vi "MeaCurr8341.vi"(10 "测试类型":u16(ring) items=["DCV", "ACV", "DCI", "ACI", "OHM", "RST", "CAP", "FRQ", "AUTO"], 11 "VISA名称":refnum<visa-resource-name>="COM1") -> (0 "错误输出":errorcluster, 2 "数值":dbl format="%#_3g")   [LabVIEW 2013]
uses:
  <vilib>/Instr/_visa.llb/VISA Flush IO Buffer Mask.ctl
  <vilib>/Instr/_visa.llb/VISA Configure Serial Port (Instr).vi
panel:
  out "响应":string
  in  "串口设置":T1={"波特率"=9600, "数据比特"=8, "奇偶"=enum."None", "停止位"=10, "流控制"=0} {"流控制" items=["无"=0, "XON/XOFF"=1, "RTS/CTS"=2, "DTR/DSR"=4]; "停止位" items=["1.0"=10, "1.5"=15, "2.0"=20]; "数据比特" min=5 max=8 step=1; "波特率" items=["75"=75, "110"=110, "134"=134, "150"=150, "300"=300, "600"=600, "1200"=1200, "1800"=1800, "2400"=2400, "4800"=4800, "7200"=7200, "9600"=9600, "14400"=14400, "19200"=19200, "28800"=28800, "38400"=38400, "56000"=56000, "57600"=57600, "115200"=115200, "128000"=128000, "230400"=230400]}
  in  "读取前延时":u32=600
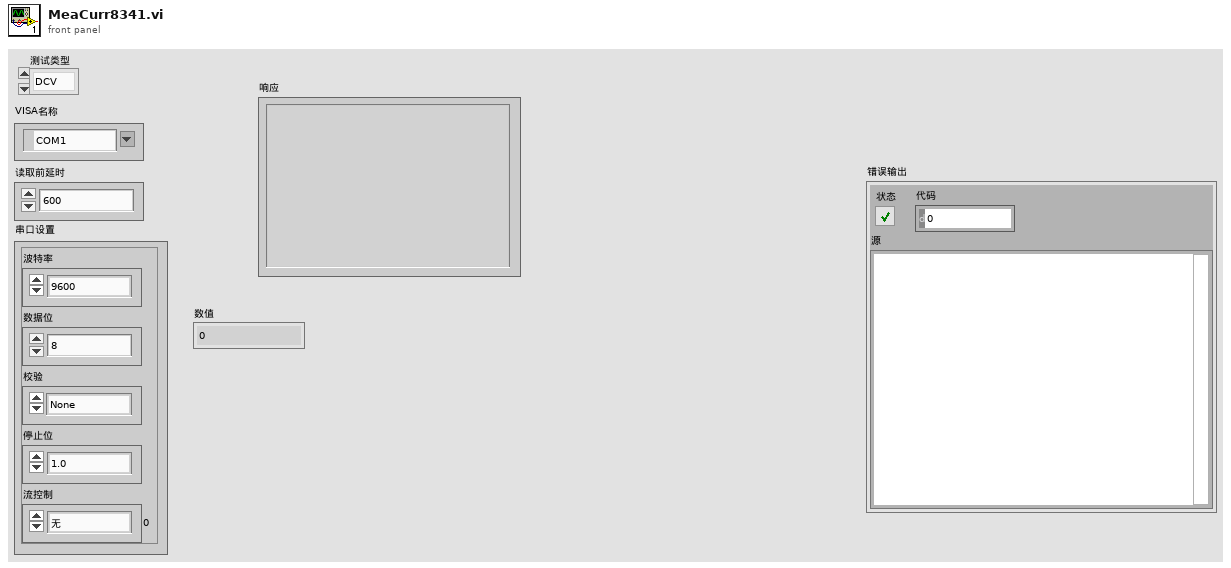
[diagram p1: front panel]
types:
  T1 = cluster{"波特率":u32, "数据比特":u16, "奇偶":enum16{"None", "Odd", "Even", "Mark", "Space"}, "停止位":u16, "流控制":u16}
  T2 = typedef "VISA Flush IO Buffer Mask.ctl" = u16
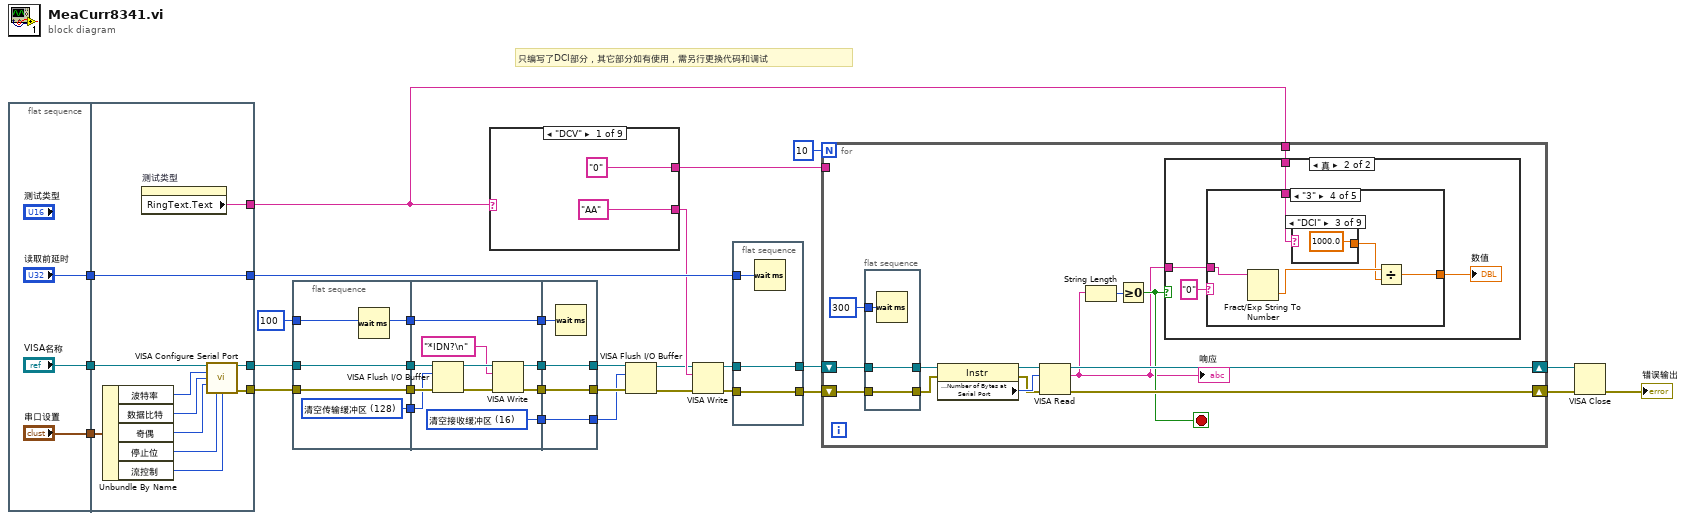
[diagram p0: block diagram]
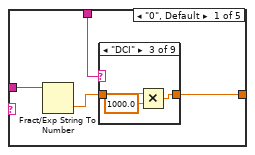
[diagram p3: hidden frame]
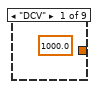
[diagram p4: hidden frame]
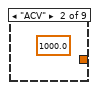
[diagram p5: hidden frame]
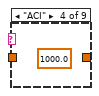
[diagram p6: hidden frame]
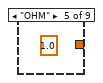
[diagram p7: hidden frame]
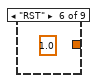
[diagram p8: hidden frame]
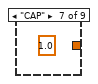
[diagram p9: hidden frame]
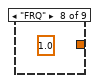
[diagram p10: hidden frame]
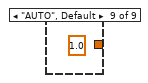
[diagram p11: hidden frame]
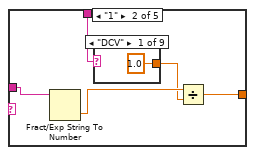
[diagram p12: hidden frame]
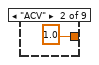
[diagram p13: hidden frame]
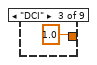
[diagram p14: hidden frame]
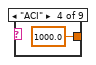
[diagram p15: hidden frame]
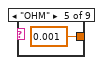
[diagram p16: hidden frame]
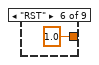
[diagram p17: hidden frame]
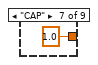
[diagram p18: hidden frame]
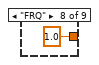
[diagram p19: hidden frame]
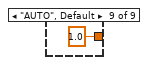
[diagram p20: hidden frame]
diagram:
  # "只编写了DCI部分，其它部分如有使用，需另行更换代码和调试"
  n1 = flat-sequence {
    tunnel: ["VISA名称"] -> w9
    tunnel: ["读取前延时"] -> w8
    tunnel: ["串口设置"] -> w7
    tunnel: [w45] -> w27
    tunnel: w9 -> [w38]
    tunnel: w8 -> [w45]
    tunnel: w7 -> [w39]
    tunnel: [w37] -> w5
    tunnel: [w36] -> w3
    tunnel: [w35] -> w2
    frame #0 {
    }
    frame #1 {
      n2 = Unbundle By Name(w39) -> ("波特率"=w40:u32, "数据比特"=w41:u16, "奇偶"=w42:enum16{"None", "Odd", "Even", "Mark", "Space"}, "停止位"=w43:u16, "流控制"=w44:u16)
      n3 = property on="测试类型" class="Ring (严格)"() -> ("RingText.Text"=w35:string)  [unwired: 2 in, 2 out]
      n4 = call-poly "VISA Configure Serial Port"("VISA resource name"=w38, "baud rate (9600)"=w40, "data bits (8)"=w41, "parity (0:none)"=w42, "stop bits (10: 1 bit)"=w43, "flow control (0:none)"=w44) -> ("VISA resource name out"=w37:refnum<visa-resource-name>, "error out"=w36:errorcluster)  [unwired: 3 in, 5 out]
    }
  }
  n5 = flat-sequence {
    tunnel: u32 100 ("读取前延时(ms)") -> [w49]
    tunnel: [w49] -> w18
    tunnel: [w48] -> w6
    tunnel: w5 -> [w48]
    tunnel: [w47] -> w4
    tunnel: w3 -> [w47]
    tunnel: [w46] -> w1
    tunnel: [w55] -> w21
    tunnel: [w56] -> w20
    tunnel: [w54] -> w19
    tunnel: w18 -> [w54]
    tunnel: [w53] -> w17
    tunnel: w6 -> [w52]
    tunnel: w4 -> [w51]
    tunnel: w1 -> [w50]
    tunnel: [w61] -> w14
    tunnel: [w62] -> w13
    tunnel: w21 -> [w62]
    tunnel: w20 -> [w61]
    tunnel: w19 -> [w63]
    tunnel: w17 -> [w60]
    tunnel: [w60] -> w12
    frame #0 {
      w46 = T2 128 items=["清空接收缓冲区"=16, "向设备写入传输缓冲区"=32, "清空接收缓冲区（无I/O）"=64, "清空传输缓冲区"=128] ("Mask")
      n6 = Wait (ms)(milliseconds to wait=w49) -> ()  [unwired: 1 out]
    }
    frame #1 {
      w53 = T2 16 items=["清空接收缓冲区"=16, "向设备写入传输缓冲区"=32, "清空接收缓冲区（无I/O）"=64, "清空传输缓冲区"=128] ("Mask")
      n7 = VISA Flush I/O Buffer(VISA resource name=w52, mask (16)=w50, error in (no error)=w51) -> (VISA resource name out=w58:refnum<visa-resource-name>, error out=w59:errorcluster)
      n8 = VISA Write(VISA resource name=w58, write buffer="*IDN?\n" ("写入缓冲区"), error in (no error)=w59) -> (VISA resource name out=w56:refnum<visa-resource-name>, error out=w55:errorcluster)  [unwired: 1 out]
    }
    frame #2 {
      n9 = Wait (ms)(milliseconds to wait=w63) -> ()  [unwired: 1 out]
    }
  }
  n10 = case shown="\"DCV\"" w2 {
    tunnel: ["AA" ("Command") "BB" ("Command") "MEAS:CURR:DC? 5e\n" "DD" ("Command") "EE" ("Command") "FF" ("Command") "GG" ("Command") "HH" ("Command") "MM" ("Command")] -> w26
    tunnel: ["0" ("Command") "1" ("Command") "3" ("Command") "4" ("Command") "6" ("Command") "F" ("Command") "7" ("Command") "8" ("Command") "M" ("Command")] -> w25
    frame "DCV" {
    }
    frame "ACV" {
    }
    frame "DCI" {
      n11 = local write "数值"(0.0 ("数值")) -> ()
    }
    frame "ACI" {
    }
    frame "OHM" {
    }
    frame "RST" {
    }
    frame "CAP" {
    }
    frame "FRQ" {
    }
    frame "AUTO", Default {
    }
  }
  n12 = VISA Flush I/O Buffer(VISA resource name=w14, mask (16)=w12, error in (no error)=w13) -> (VISA resource name out=w10:refnum<visa-resource-name>, error out=w11:errorcluster)
  n13 = VISA Write(VISA resource name=w10, write buffer=w26, error in (no error)=w11) -> (VISA resource name out=w16:refnum<visa-resource-name>, error out=w15:errorcluster)  [unwired: 1 out]
  n14 = flat-sequence {
    tunnel: [w83] -> w29
    tunnel: [w84] -> w28
    tunnel: w27 -> [w85]
    tunnel: w16 -> [w84]
    tunnel: w15 -> [w83]
    frame #0 {
      n15 = Wait (ms)(milliseconds to wait=w85) -> ()  [unwired: 1 out]
    }
  }
  n16 = for {
    N: 10 -> [_]
    tunnel: w25 -> [_]
    tunnel: w2 -> [w96]
    shift-right: [w98] -> w30
    shift-left: w28 -> [w95]
    shift-right: [w99] -> w31
    shift-left: w29 -> [w93]
    stop <- w90 stop-if-true
    n17 = flat-sequence {
      tunnel: w93 -> [w101]
      tunnel: [w101] -> w92
      tunnel: w95 -> [w100]
      tunnel: [w100] -> w94
      tunnel: u32 300 ("读取前延时(ms)") -> [w102]
      frame #0 {
        n18 = Wait (ms)(milliseconds to wait=w102) -> ()  [unwired: 1 out]
      }
    }
    n19 = property class="Instr"(reference=w94, error in=w92) -> (reference out=w89:refnum<visa-resource-name>, error out=w88:errorcluster, "Serial Settings:Number of Bytes at Serial Port"=w97:u32)
    n20 = VISA Read(VISA resource name=w89, byte count=w97, error in (no error)=w88) -> (VISA resource name out=w98:refnum<visa-resource-name>, read buffer=w86:string, error out=w99:errorcluster)  [unwired: 1 out]
    "响应" <- w86
    n21 = String Length(string=w86) -> (length=w87:i32)
    n22 = Greater Or Equal To 0?(x=w87) -> (x >= 0?=w90:bool)
    n23 = case shown="真" w90 {
      tunnel: w86 -> [_ w103]
      tunnel: w96 -> [_ w106]
      frame False {
      }
      frame True {
        n24 = case shown="\"3\"" "0" {
          tunnel: w103 -> [w110 w118 w132 w146 w160]
          tunnel: w106 -> [w109 w117 w131 w145 w159]
          tunnel: [w108 w114 w128 w142 w156] -> w105
          frame "0", Default {
            n25 = Fract/Exp String To Number(string=w110) -> (number=w107:dbl)  [unwired: 3 in, 1 out]
            n26 = case shown="\"DCI\"" w109 {
              tunnel: [_ _ w111 _ _ _ _ _ _] -> w108
              tunnel: w107 -> [_ _ w113 _ _ _ _ _ _]
              frame "DCV" {
                (unwired) 1000.0
              }
              frame "ACV" {
                (unwired) 1000.0
              }
              frame "DCI" {
                n27 = Multiply(x=w113, y=1000.0) -> (x*y=w111:dbl)
              }
              frame "ACI" {
                (unwired) 1000.0
              }
              frame "OHM" {
                (unwired) 1.0
              }
              frame "RST" {
                (unwired) 1.0
              }
              frame "CAP" {
                (unwired) 1.0
              }
              frame "FRQ" {
                (unwired) 1.0
              }
              frame "AUTO", Default {
                (unwired) 1.0
              }
            }
          }
          frame "1" {
            n28 = Fract/Exp String To Number(string=w118) -> (number=w116:dbl)  [unwired: 3 in, 1 out]
            n29 = case shown="\"DCV\"" w117 {
              tunnel: [1.0 1.0 1.0 1000.0 0.001 1.0 1.0 1.0 1.0] -> w115
              frame "DCV" {
              }
              frame "ACV" {
              }
              frame "DCI" {
              }
              frame "ACI" {
              }
              frame "OHM" {
              }
              frame "RST" {
              }
              frame "CAP" {
              }
              frame "FRQ" {
              }
              frame "AUTO", Default {
              }
            }
            n30 = Divide(x=w116, y=w115) -> (x/y=w114:dbl)
          }
          frame "2" {
            n31 = Fract/Exp String To Number(string=w132) -> (number=w130:dbl)  [unwired: 3 in, 1 out]
            n32 = case shown="\"DCV\"" w131 {
              tunnel: [1.0 1.0 1000.0 1000.0 0.001 1.0 1.0 1.0 1.0] -> _
              frame "DCV" {
              }
              frame "ACV" {
              }
              frame "DCI" {
              }
              frame "ACI" {
              }
              frame "OHM" {
              }
              frame "RST" {
              }
              frame "CAP" {
              }
              frame "FRQ" {
              }
              frame "AUTO", Default {
              }
            }
            n33 = Multiply(x=w130, y=1000.0) -> (x*y=w128:dbl)
          }
          frame "3" {
            n34 = Fract/Exp String To Number(string=w146) -> (number=w144:dbl)  [unwired: 3 in, 1 out]
            n35 = case shown="\"DCI\"" w145 {
              tunnel: [1.0 1.0 1000.0 1000.0 0.001 1.0 1.0 1.0 1.0] -> w143
              frame "DCV" {
              }
              frame "ACV" {
              }
              frame "DCI" {
              }
              frame "ACI" {
              }
              frame "OHM" {
              }
              frame "RST" {
              }
              frame "CAP" {
              }
              frame "FRQ" {
              }
              frame "AUTO", Default {
              }
            }
            n36 = Divide(x=w144, y=w143) -> (x/y=w142:dbl)
          }
          frame "4" {
            n37 = Fract/Exp String To Number(string=w160) -> (number=w158:dbl)  [unwired: 3 in, 1 out]
            n38 = case shown="\"DCI\"" w159 {
              tunnel: [1.0 1.0 1000.0 1000.0 1e-06 1.0 1.0 1.0 1.0] -> w157
              frame "DCV" {
              }
              frame "ACV" {
              }
              frame "DCI" {
              }
              frame "ACI" {
              }
              frame "OHM" {
              }
              frame "RST" {
              }
              frame "CAP" {
              }
              frame "FRQ" {
              }
              frame "AUTO", Default {
              }
            }
            n39 = Divide(x=w158, y=w157) -> (x/y=w156:dbl)
          }
        }
        "数值" <- w105
      }
    }
  }
  n40 = VISA Close(VISA resource name=w30, error in (no error)=w31) -> (error out=→"错误输出":errorcluster)
